vi "Charger_Charge Enabled.vi"(6 "Stop Refnum":refnum<vi>, 7 "Status Refnum":T1, 8 "error in":errorcluster) -> (0 "error out":errorcluster)   [LabVIEW 2020]
uses:
  Charger_Status Refnum.ctl
  Drivers/Charger Test Set/Charger_Input Control.ctl
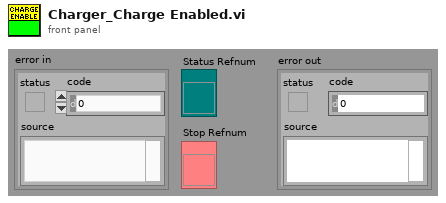
[diagram p1: front panel]
types:
  T1 = typedef "Charger_Status Refnum.ctl" = refnum<vi>
  T2 = typedef "Charger_Input Control.ctl" = cluster{"address":refnum<visa-resource-name>, "position":i32, "setpoint":dbl}
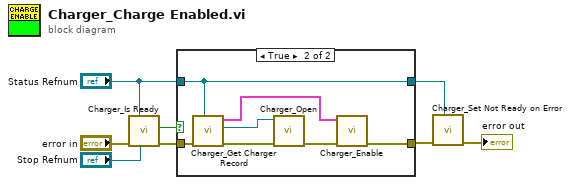
[diagram p0: block diagram]
diagram:
  n1 = call "Charger_Is Ready.vi"("Stop Refnum"="Stop Refnum", "Status Refnum"="Status Refnum", "error in"="error in") -> ("error out"=w6:errorcluster, "ready"=w5:bool)  [unwired: 7 in]
  n2 = case shown="True" w5 {
    tunnel: [w10 w11] -> w3
    tunnel: "Status Refnum" -> [w9 w12]
    tunnel: w6 -> [w10 w15]
    tunnel: [w9 w12] -> w2
    frame False {
    }
    frame True {
      n3 = call "Charger_Get Charger Record.vi"("Status Refnum"=w12, "error in"=w15) -> ("error out"=w14:errorcluster, "address"=w16:refnum<visa-resource-name>, "Charger Inputs"=w13:T2)  [unwired: 3 in, 2 out]
      n4 = call "Charger_Open.vi"("error in"=w14, "Charger COM port"=w16) -> ("error out"=w17:errorcluster)  [unwired: 5 in]
      n5 = call "Charger_Enable.vi"("error in"=w17, "Charger"=w13) -> ("error out"=w11:errorcluster)  [unwired: 7 in]
    }
  }
  n6 = call "Charger_Set Not Ready on Error.vi"("Status Refnum"=w2, "error in"=w3) -> ("error out"=→"error out":errorcluster)  [unwired: 7 in, 1 out]
